vi "Pre Init.vi"(8 "error in (no error)":errorcluster, 11 "Mag Lab Measure Base in":refnum<class "Mag Lab Measure Base.lvclass">) -> (0 "error out":errorcluster, 3 "Mag Lab Measure Base out":refnum<class "Mag Lab Measure Base.lvclass">)   [LabVIEW 2015, in "Mag Lab Measure Base.lvclass"]
uses:
  Mag Lab Measure Base.lvclass
  Mag Lab Root/Mag Lab Root.lvclass/Mag Lab Root.ctl
  Mag Lab Measure Base.lvclass/Mag Lab Measure Base.ctl
  Mag Lab Root/Mag Lab Root.lvclass
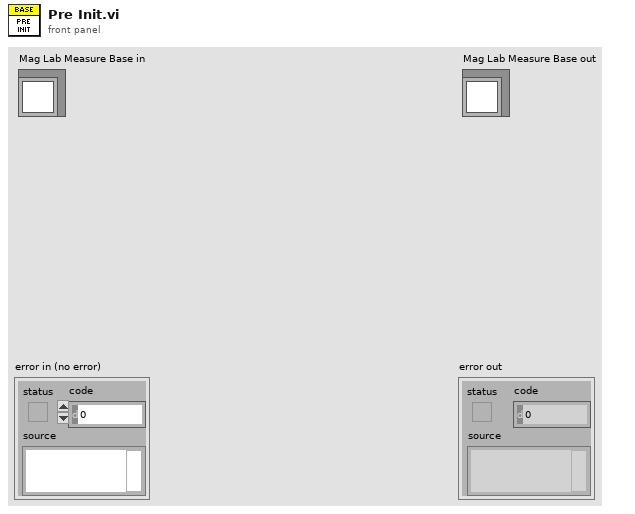
[diagram p1: front panel]
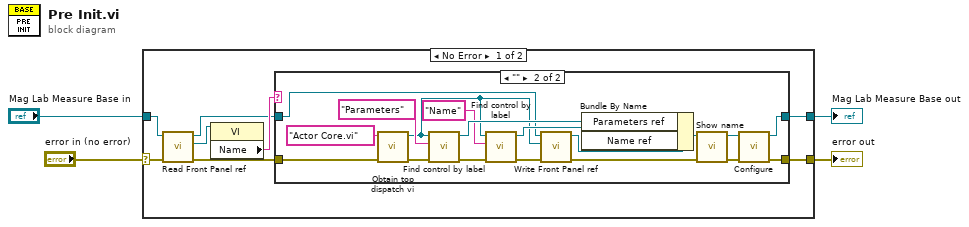
[diagram p0: block diagram]
diagram:
  n1 = case shown="No Error" "error in (no error)" {
    selector: "error in (no error)" -> [w6 w34]
    tunnel: [w10 w34] -> w3
    tunnel: [w11 w33] -> w1
    tunnel: "Mag Lab Measure Base in" -> [w9 w33]
    frame No Error {
      n2 = call "Read Front Panel ref.vi"("error in (no error)"=w6, "Mag Lab Root in"=w9) -> ("error out"=w5:errorcluster, "Front Panel ref"=w7:refnum<vi>, "Mag Lab Root out"=w8:refnum<class "Mag Lab Measure Base.lvclass">)  [unwired: 7 in]
      n3 = property class="VI"(reference=w7) -> ("Name"=w12:string)  [unwired: 1 in, 2 out]
      n4 = case shown="\"\"" w12 {
        tunnel: w8 -> [w14 w19]
        tunnel: w5 -> [w13 w31]
        tunnel: [w14 w30] -> w11
        tunnel: [w13 w29] -> w10
        frame Default {
        }
        frame "" {
          n5 = call "Obtain top dispatch vi.vi"("Error In"=w31, "VI name"="Actor Core.vi") -> ("Error Out"=w20:errorcluster, "vi reference"=w18:refnum<vi>)  [unwired: 7 in, 1 out]
          n6 = call "Find control by label.vi"("error in (no error)"=w20, "Label"="Parameters", "VI ref"=w18) -> ("error out"=w27:errorcluster, "Control out"=w26:refnum<vi>)  [unwired: 6 in, 1 out]
          n7 = call "Find control by label.vi"("error in (no error)"=w27, "Label"="Name", "VI ref"=w18) -> ("error out"=w17:errorcluster, "Control out"=w25:refnum<vi>)  [unwired: 6 in, 1 out]
          n8 = call "Write Front Panel ref.vi"("error in (no error)"=w17, "Front Panel ref"=w18, "Mag Lab Root in"=w19) -> ("error out"=w16:errorcluster, "Mag Lab Root out"=w15:refnum<class "Mag Lab Measure Base.lvclass">)  [unwired: 7 in]
          n9 = Bundle By Name(cluster=w15, "Parameters ref"=w26, "Name ref"=w25) -> (w22:refnum<class "Mag Lab Measure Base.lvclass">)
          n10 = call "Show name.vi"("error in (no error)"=w16, "Mag Lab Measure Base in"=w22) -> ("error out"=w24:errorcluster, "Mag Lab Measure Base out"=w23:refnum<class "Mag Lab Measure Base.lvclass">)  [unwired: 8 in]
          n11 = call-dynamic "Configure.vi"("error in (no error)"=w24, "Mag Lab Root in"=w23) -> ("error out"=w29:errorcluster, "Mag Lab Root out"=w30:refnum<class "Mag Lab Measure Base.lvclass">)  [unwired: 8 in]
        }
      }
    }
    frame Error {
    }
  }
  "error out" <- w3
  "Mag Lab Measure Base out" <- w1
